vi "Save config.vi"(6 "VI ref":refnum<vi>, 7 "Control names":string[](array[string]), 8 "error in (no error)":errorcluster, 10 "Graph_refs":T1, 11 "configuration file path":path) -> (0 "error out":errorcluster)   [LabVIEW 2018]
uses:
  Scope/controls/Graph_references.ctl
  Scope/controls/graph_controls.ctl
  <vilib>/Utility/config.llb/NI_LVConfig.lvlib
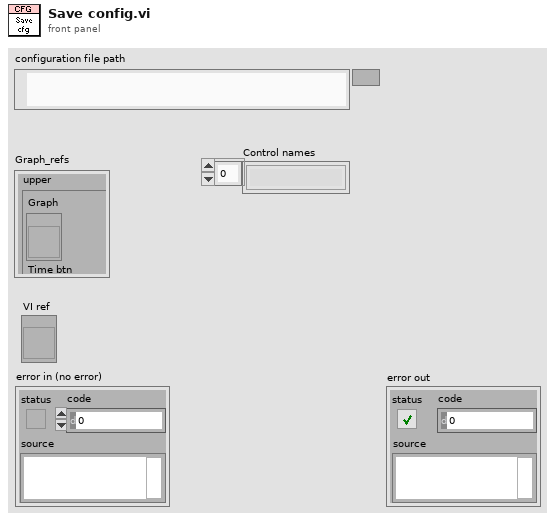
[diagram p1: front panel]
types:
  T1 = typedef "Graph_references.ctl" = cluster{"upper":T2, "lower":T2, "Freq graph":refnum<vi>, "Adaptive FF graph":refnum<vi>}
  T2 = typedef "graph_controls.ctl" = cluster{"Graph":refnum<vi>, "Time btn":refnum<vi>, "Amplitude btn":refnum<vi>, "Chart":refnum<vi>}
  T3 = typedef "NI_LVConfig.lvlib/Config Data RefNum.ctl" = refnum<k1>
  T4 = typedef "Plot visibility.ctl" = cluster{"Visible":bool[], "Name":string}
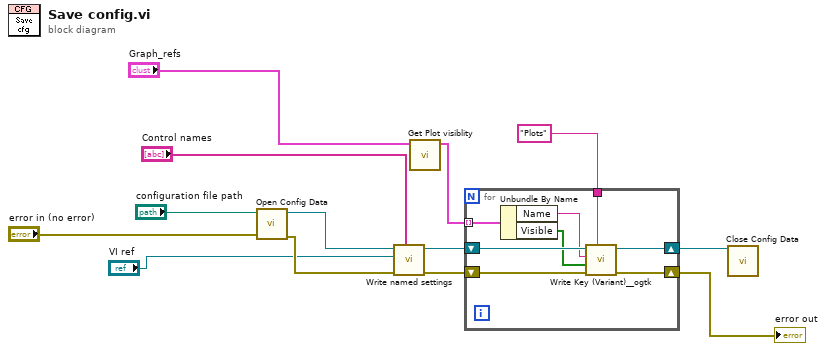
[diagram p0: block diagram]
diagram:
  n1 = call <vilib>:"Open Config Data.vi"("error in (no error)"="error in (no error)", "configuration file path"="configuration file path") -> ("error out"=w11:errorcluster, "refnum"=w13:T3)  [unwired: 7 in, 1 out]
  n2 = call "Write named settings.vi"("Names"="Control names", "error in (no error)"=w11, "VI ref"="VI ref", "refnum"=w13) -> ("error out"=w7:errorcluster, "refnum out"=w8:T3)  [unwired: 6 in]
  n3 = call "Get Plot visiblity.vi"("Graph_refs"="Graph_refs") -> ("Plot visibility"=w9:T4[])  [unwired: 10 in]
  n4 = for {
    tunnel: w9 -> [w18] mode=indexing
    shift-right: [w19] -> w6
    shift-left: w8 -> [w21]
    tunnel: "Plots" -> [w15]
    shift-right: [w14] -> w4
    shift-left: w7 -> [w20]
    n5 = Unbundle By Name(w18) -> ("Name"=w16:string, "Visible"=w17:bool[])
    n6 = call <userlib>:"Write Key (Variant)__ogtk.vi"("section"=w15, "error in (no error)"=w20, "key-value"=w17, "key (optional)"=w16, "refnum"=w21) -> ("error out"=w14:errorcluster, "refnum out"=w19:T3)  [unwired: 5 in]
  }
  "error out" <- w4
  n7 = call <vilib>:"Close Config Data.vi"("refnum"=w6) -> ()  [unwired: 9 in, 2 out]
